vi "Miso Logic 128-bit.vi"(0 "MISO":bool, 5 "sample MISO":bool, 7 "controller interface":T1) -> (4 "read data":bool[](array[boolean]))   [LabVIEW 2015, in "SPI API.lvlib"]
doc: "This VI captures a single bit of MISO data to for the read data word."
uses:
  Controls/Controller Interface.ctl
  SPI API.lvlib
panel:
  # "This VI captures a single bit of MISO data to for the read data word."
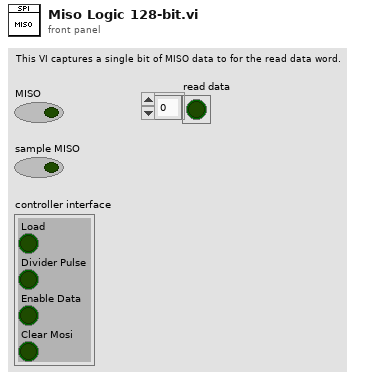
[diagram p1: front panel]
types:
  T1 = typedef "SPI API.lvlib/Controller Interface.ctl" = cluster{"Load":bool, "Divider Pulse":bool, "Enable Data":bool, "Clear Mosi":bool}
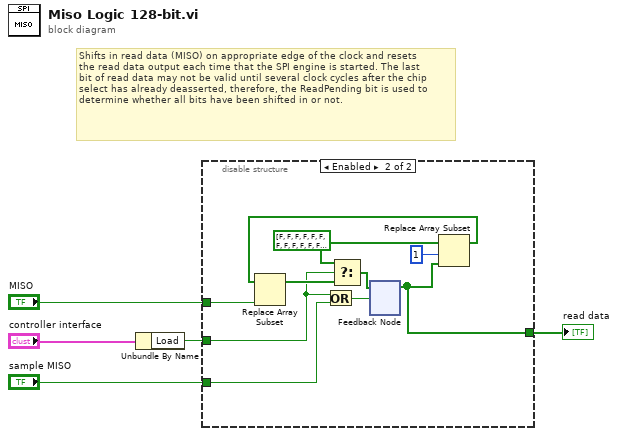
[diagram p0: block diagram]
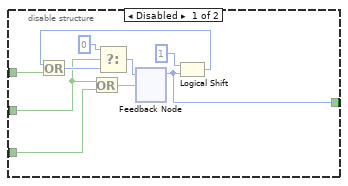
[diagram p2: hidden frame]
diagram:
  # "Shifts in read data (MISO) on appropriate edge of the clock and resets\nthe read data output each time that the SPI engine is started. The last\nbit of read data may not be valid until several clock cycles after the chip select has already deasserted, therefore, the ReadPending bit is used to determine whether all bits have been shifted in or not."
  n1 = Unbundle By Name("controller interface") -> ("Load"=w5:bool)
  n2 = disable-structure shown="Enabled" {
    disable-tunnel: [w14 w16] -> w1
    disable-tunnel: "MISO" -> [w13 w20]
    disable-tunnel: w5 -> [w7 w21]
    disable-tunnel: "sample MISO" -> [w6 w23]
    frame Disabled {
      n3 = Or(x=w7, y=w6) -> (x .or. y?=w11:bool)
      n4 = feedback #1() -> (w14:u64)  [unwired: 1 in]
      n5 = Logical Shift(y=i16 1, x=w14) -> (x << y=w12:u64)
      n6 = Or(x=w12, y=w13) -> (x .or. y?=w10:u64)
      n7 = Select(t=u64 0, s=w7, f=w10) -> (s? t:f=w9:u64)
      n8 = feedback-in #1(w9, w11) -> ()
    }
    frame Enabled {
      w19 = bool[] [FALSE, FALSE, FALSE, FALSE, FALSE, FALSE, FALSE, FALSE, FALSE, FALSE, FALSE, FALSE, FALSE, FALSE, FALSE, FALSE, FALSE, FALSE, FALSE, FALSE, FALSE, FALSE, FALSE, FALSE, FALSE, FALSE, FALSE, FALSE, FALSE, FALSE, FALSE, FALSE, FALSE, FALSE, FALSE, FALSE, FALSE, FALSE, FALSE, FALSE, FALSE, FALSE, FALSE, FALSE, FALSE, FALSE, FALSE, FALSE, FALSE, FALSE, FALSE, FALSE, FALSE, FALSE, FALSE, FALSE, FALSE, FALSE, FALSE, FALSE, FALSE, FALSE, FALSE, FALSE, FALSE, FALSE, FALSE, FALSE, FALSE, FALSE, FALSE, FALSE, FALSE, FALSE, FALSE, FALSE, FALSE, FALSE, FALSE, FALSE, FALSE, FALSE, FALSE, FALSE, FALSE, FALSE, FALSE, FALSE, FALSE, FALSE, FALSE, FALSE, FALSE, FALSE, FALSE, FALSE, FALSE, FALSE, FALSE, FALSE, FALSE, FALSE, FALSE, FALSE, FALSE, FALSE, FALSE, FALSE, FALSE, FALSE, FALSE, FALSE, FALSE, FALSE, FALSE, FALSE, FALSE, FALSE, FALSE, FALSE, FALSE, FALSE, FALSE, FALSE, FALSE, FALSE, FALSE, FALSE]
      n9 = Or(x=w21, y=w23) -> (x .or. y?=w25:bool)
      n10 = feedback #2() -> (w16:bool[])  [unwired: 1 in]
      n11 = Replace Array Subset(array=w19, new element=w16, index=1) -> (w17:bool[])
      n12 = Replace Array Subset(array=w17, new element=w20) -> (w22:bool[])  [unwired: 1 in]
      n13 = Select(t=w19, s=w21, f=w22) -> (s? t:f=w24:bool[])
      n14 = feedback-in #2(w24, w25) -> ()
    }
  }
  "read data" <- w1
